vi "lookfordata_i32.vi"(1 "string (in)":string, 2 "Header":string) -> (4 "offset past match":i32, 6 "output number":i32, 7 "output string":string)   [LabVIEW 8.6]
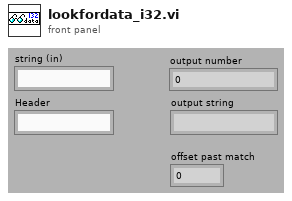
[diagram p1: front panel]
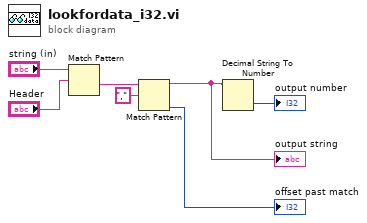
[diagram p0: block diagram]
diagram:
  n1 = Match Pattern(string="string (in)", regular expression="Header") -> (after substring=w4:string)  [unwired: 4 out]
  n2 = Match Pattern(string=w4, regular expression=",") -> (before substring=w3:string, offset past match=→"offset past match":i32)  [unwired: 3 out]
  "output string" <- w3
  n3 = Decimal String To Number(string=w3) -> (number=→"output number":i32)  [unwired: 3 out]
